vi "Robot Main.vi"() -> ()   [LabVIEW 2016]
doc: "This VI implements the framework and scheduler for your robotics program. It should not be necessary to modify the framework. You are expected to add your code to the VIs called from Robot Main - the ones located in the Team Code folder within the project."
uses:
  <vilib>/Rock Robotics/WPI/Camera/WPI_CameraImageSize.ctl
  <vilib>/Rock Robotics/WPI/ThirdParty/Sensors/navX/_TypeDefs/FRIC_navX_DeviceNumbersTypeDef.ctl
  <vilib>/Rock Robotics/SystemInterfaces/i2clib/i2c_bus.ctl
  <vilib>/Rock Robotics/WPI/ThirdParty/Sensors/navX/_Processing Loop/FRIC_navX_Internal_I2C_ProcessingLoop.vi
  Robot Global Data.vi
  AutoaimVar.vi
panel:
  out "Thermometer":dbl(slide) scale=-720.0..720.0
  in  "New Gyro":bool
  in  "Image Size":T1=enum."160x120"
  in  "Enable Vision":bool=TRUE
  in  "Finish":bool
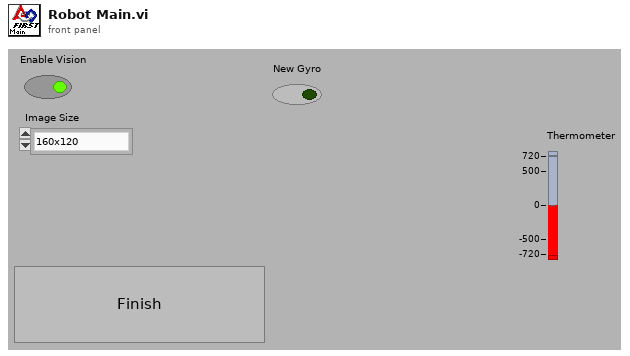
[diagram p1: front panel]
types:
  T1 = typedef "WPI_CameraImageSize.ctl" = enum16{"640x480", "320x240", "160x120", "Custom"}
  T2 = typedef "i2c_bus.ctl" = enum16{"I2C On-Board", "I2C MXP", "Invalid"}
  T3 = typedef "FRIC_navX_DeviceNumbersTypeDef.ctl" = enum16{"Dev0", "Dev1", "Dev2", "Dev3"}
  T4 = typedef "WPI_DriverStationMatch Info.ctl" = cluster{"Autonomous Elapsed Seconds":dbl, "TeleOp Elapsed Seconds":dbl, "Disabled Elapsed Seconds":dbl, "Visited Autonomous":bool, "Visited TeleOp":bool, "Visited Disabled":bool, "Autonomous Settings":cluster{"Autonomous Style":enum16{"Iterative", "Independent"}, "VI Refnum":refnum<vi>}}
  T5 = typedef "WPI_DriverStationDerivedRobotMode.ctl" = enum16{"Init", "Execute", "Stop"}
  T6 = typedef "WPI_DriverStationRobotMode2.ctl" = enum16{"Autonomous Disabled", "Autonomous Enabled", "Teleop Disabled", "Teleop Enabled", "Disconnected", "Finish", "Test Disabled", "Test Enabled", "Emergency Stopped"}
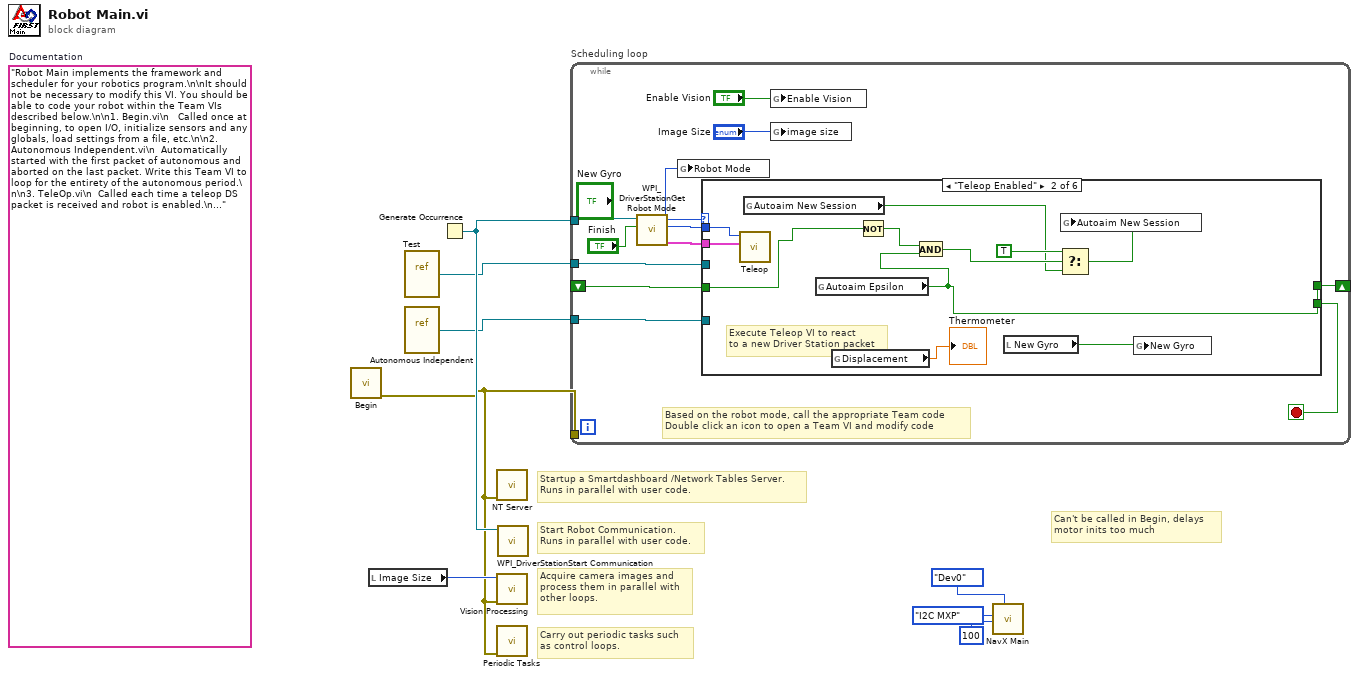
[diagram p0: block diagram]
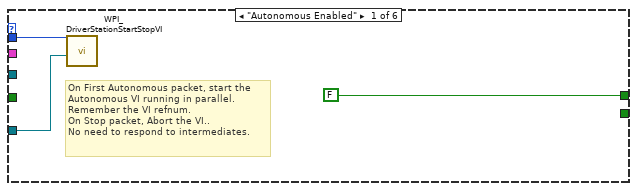
[diagram p2: hidden frame]
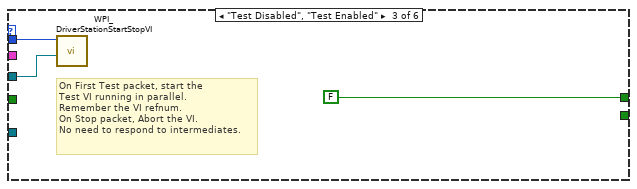
[diagram p3: hidden frame]
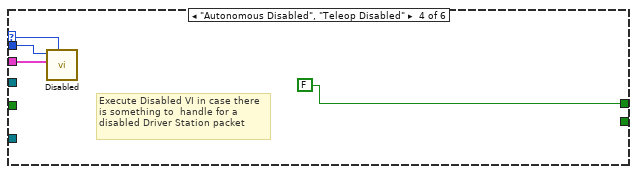
[diagram p4: hidden frame]
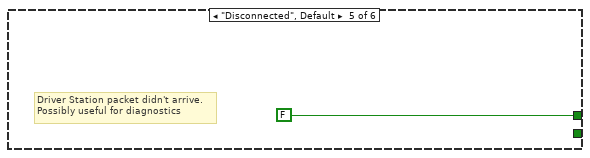
[diagram p5: hidden frame]
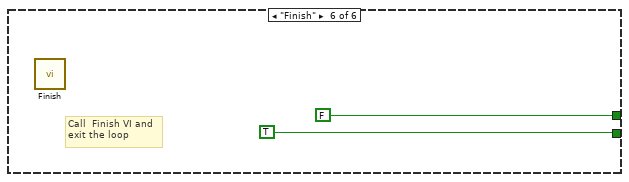
[diagram p6: hidden frame]
diagram:
  (unwired) "Robot Main implements the framework and scheduler for your robotics program.\n\nIt should not be necessary to modify this VI. You should be able to code your robot within the Team VIs described below.\n\n1. Begin.vi\n   Called once at beginning, to open I/O, initialize sensors and any globals, load settings from a file, etc.\n\n2. Autonomous Independent.vi\n  Automatically started with the first packet of autonomous and aborted on the last packet. Write this Team VI to loop for the entirety of the autonomous period.\n\n3. TeleOp.vi\n  Called each time a teleop DS packet is received and robot is enabled.\n\n4. Disabled.vi\n  Called each time a packet is received and the robot is disabled.\n\n5. Test.vi\n  Called Automatically started with the first test packet and aborted on the last. Modify this VI to carry out robot and sensor validation tests.\n\n6. Vision.vi\n  A parallel loop that acquires and processes camera images.\n\n7. PeriodicTasks.vi\n  Parallel loops running at user-defined rates.\n\n8. Finish.vi\n  Called before exiting, so you can save data, clean up I/O, etc.\n"  # Documentation
  # "Can't be called in Begin, delays \nmotor inits too much"
  # "Startup a Smartdashboard /Network Tables Server.\nRuns in parallel with user code."
  # "Carry out periodic tasks such\nas control loops."
  # "Acquire camera images and\nprocess them in parallel with\nother loops."
  # "Start Robot Communication.\nRuns in parallel with user code."
  n1 = call "Begin.vi"() -> ("error out"=w1:errorcluster)  [unwired: 2 in, 9 out]
  n2 = local read "Image Size"() -> (w5:T1)
  n3 = vi-ref "Test.vi"() -> (w6:refnum<vi>)
  n4 = vi-ref "Autonomous Independent.vi"() -> (w7:refnum<vi>)
  n5 = Generate Occurrence() -> (w8:refnum<k4>)
  n6 = call <vilib>:"NT Server.vi"("error in (no error)"=w1) -> ()  [unwired: 11 in]
  n7 = call "Vision Processing.vi"("error in (no error)"=w1, "Image Size"=w5) -> ()  [unwired: 6 out]
  n8 = call "Periodic Tasks.vi"("error in"=w1) -> ()  [unwired: 1 in, 10 out]
  n9 = call <vilib>:"WPI_DriverStationStart Communication.vi"("occurrence"=w8) -> ()  [unwired: 1 in, 10 out]
  n10 = while "Scheduling loop" {
    tunnel: w8 -> [w19]
    tunnel: w1 -> [_]
    tunnel: w7 -> [w14]
    tunnel: w6 -> [w12]
    shift-right: [w10] -> _
    shift-left: _ -> [w9]
    stop <- w16 stop-if-true
    # "Based on the robot mode, call the appropriate Team code\nDouble click an icon to open a Team VI and modify code"
    n11 = call <vilib>:"WPI_DriverStationGet Robot Mode.vi"("Finish"="Finish", "DS Occurrence"=w19) -> ("Match Info out"=w17:T4, "Call Context"=w20:T5, "Robot Mode"=w11:T6)  [unwired: 7 out]
    n12 = global write "Robot Global Data.vi" "Robot Mode"(w11) -> ()
    n13 = case shown="\"Teleop Enabled\"" w11 {
      selector: w11 -> [_ _ _ w39 _ _]
      tunnel: w20 -> [w23 w34 w37 w41 _ _]
      tunnel: w17 -> [_ w33 _ w40 _ _]
      tunnel: [_ _ _ _ _ TRUE] -> w16
      tunnel: w14 -> [w22 _ _ _ _ _]
      tunnel: w12 -> [_ _ w36 _ _ _]
      tunnel: [FALSE ("Autoaim Epsilon") w28 FALSE ("Autoaim Epsilon") FALSE FALSE ("Autoaim Epsilon") FALSE ("Autoaim Epsilon")] -> w10
      tunnel: w9 -> [_ w30 _ _ _ _]
      frame "Autonomous Enabled" {
        # "On First Autonomous packet, start the\nAutonomous VI running in parallel.\nRemember the VI refnum.\nOn Stop packet, Abort the VI..\nNo need to respond to intermediates."
        n14 = call <vilib>:"WPI_DriverStationStartStopVI.vi"("VI in"=w22, "Call Context"=w23) -> ()  [unwired: 10 in]
      }
      frame "Teleop Enabled" {
        # "Execute Teleop VI to react\nto a new Driver Station packet"
        n15 = call "Teleop.vi"("Match Info"=w33, "Call Context"=w34) -> ()  [unwired: 1 in, 9 out]
        n16 = global read "AutoaimVar.vi" "Autoaim New Session"() -> (w26:bool)
        n17 = global read "AutoaimVar.vi" "Autoaim Epsilon"() -> (w28:bool)
        n18 = global read "Robot Global Data.vi" "Displacement"() -> (→"Thermometer":dbl)
        n19 = Not(x=w30) -> (.not. x?=w29:bool)
        n20 = And(x=w29, y=w28) -> (x .and. y?=w27:bool)
        n21 = local read "New Gyro"() -> (w25:bool)
        n22 = Select(t=TRUE, s=w27, f=w26) -> (s? t:f=w31:bool)
        n23 = global write "AutoaimVar.vi" "Autoaim New Session"(w31) -> ()
        n24 = global write "Robot Global Data.vi" "New Gyro"(w25) -> ()
      }
      frame "Test Disabled", "Test Enabled" {
        # "On First Test packet, start the\nTest VI running in parallel.\nRemember the VI refnum.\nOn Stop packet, Abort the VI.\nNo need to respond to intermediates."
        n25 = call <vilib>:"WPI_DriverStationStartStopVI.vi"("VI in"=w36, "Call Context"=w37) -> ()  [unwired: 10 in]
      }
      frame "Autonomous Disabled", "Teleop Disabled" {
        # "Execute Disabled VI in case there\nis something to  handle for a\ndisabled Driver Station packet"
        n26 = call "Disabled.vi"("Robot Mode"=w39, "Match Info"=w40, "Call Context"=w41) -> ()  [unwired: 1 in, 8 out]
      }
      frame "Disconnected", Default {
        # "Driver Station packet didn't arrive.\nPossibly useful for diagnostics"
      }
      frame "Finish" {
        # "Call  Finish VI and\nexit the loop"
        n27 = call "Finish.vi"() -> ()  [unwired: 1 in, 7 out]
      }
    }
    n28 = global write "Robot Global Data.vi" "Enable Vision"("Enable Vision") -> ()
    n29 = global write "Robot Global Data.vi" "image size"("Image Size") -> ()
  }
  n30 = call-poly <vilib>:"NavX Main.vi"("Device Number"=FRIC_navX_DeviceNumbersTypeDef."Dev0", "I2C Bus"=i2c_bus."I2C MXP", "Rate (4Hz-200Hz)"=u8 100) -> ()  [unwired: 9 in]
